vi "Tag Names.vi"(11 "Process Name":string) -> (3 "Pump Module Tag Names":T1, 4 "All Boolean Tags":string[](array[string]), 5 "All  Numeric Tags":string[](array[string]))   [LabVIEW 2018, in "TCU Module.lvlib" / "TCU Module Engine.lvlib"]
uses:
  TCU Module Engine.lvlib
  TCU Module Tag Names Cluster.ctl
  TCU Module.lvlib
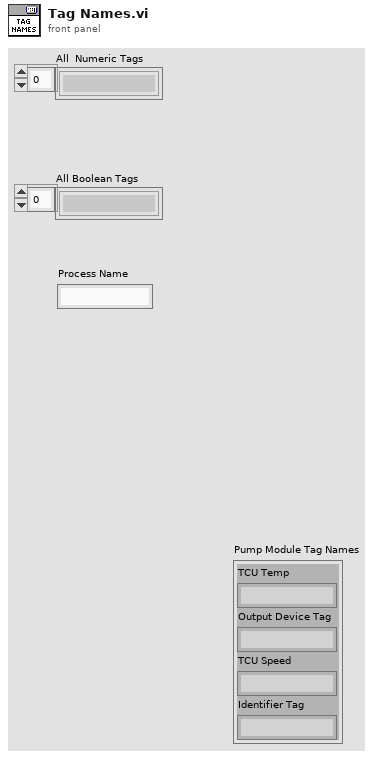
[diagram p1: front panel]
types:
  T1 = typedef "TCU Module.lvlib/TCU Module Tag Names Cluster.ctl" = cluster{"TCU Temp":string, "Output Device Tag":string, "TCU Speed":string, "Identifier Tag":string}
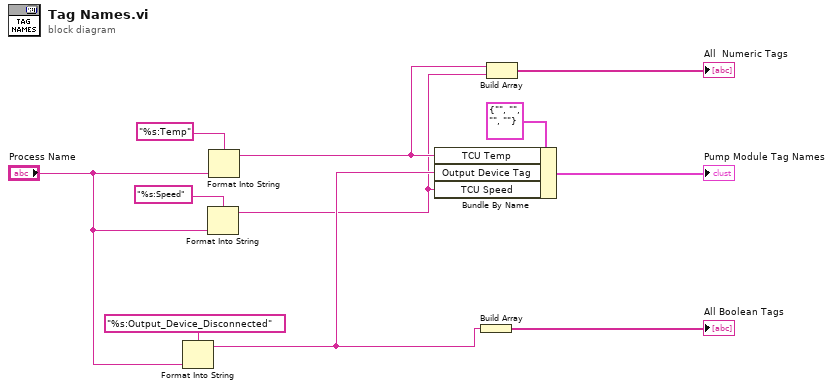
[diagram p0: block diagram]
diagram:
  n1 = Format Into String(format string="%s:Output_Device_Disconnected", "Process Name") -> (resulting string=w11:string)  [unwired: 2 in, 1 out]
  n2 = Format Into String(format string="%s:Speed", "Process Name") -> (resulting string=w1:string)  [unwired: 2 in, 1 out]
  n3 = Format Into String(format string="%s:Temp", "Process Name") -> (resulting string=w5:string)  [unwired: 2 in, 1 out]
  n4 = Bundle By Name(cluster=T1 {"TCU Temp"="", "Output Device Tag"="", "TCU Speed"="", "Identifier Tag"=""} ("Feed Module Tag Names"), "TCU Temp"=w5, "Output Device Tag"=w11, "TCU Speed"=w1) -> (→"Pump Module Tag Names":T1)
  n5 = Build Array(w11) -> (→"All Boolean Tags":string[])
  n6 = Build Array(w5, w1) -> (→"All  Numeric Tags":string[])
